vi "api_mqttInit.vi"(0 "client":string="LabVIEW_MQTT_Client", 5 "broker":T3={"address"="localhost", "port"=1883, "connTimeout"=2000, "writeTimeout"=2000, "readTimeout"=2000, "subTimeout"=30000}, 7 "connFlags":T2={"reserved"=FALSE, "clean session"=TRUE, "will flag"=TRUE, "willQOS"=enum."At most once", "will retain"=FALSE, "password"=FALSE, "user name"=FALSE}, 9 "User Info":T1={"User Name"="User", "Password"="password"}, 11 "error in (no error)":errorcluster) -> (4 "mqtt.lvclass out":refnum<class "mqtt.lvclass">, 10 "MQTT event":refnum<user-event>, 15 "error out":errorcluster)   [LabVIEW 2018, in "labview-mqtt.lvlib" / "mqtt.lvclass"]
uses:
  mqtt.lvclass
  mqttTypedef/mqttBroker.ctl
  mqttTypedef/mqttConnectionFlags.ctl
  mqttTypedef/mqttWillInformation.ctl
  mqttTypedef/mqttRXsubscriptionEventData.ctl
  mqtt.lvclass/mqtt.ctl
  labview-mqtt.lvlib
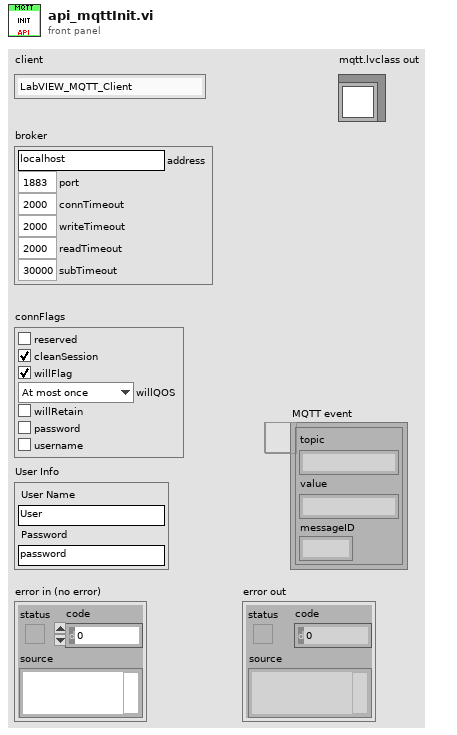
[diagram p1: front panel]
types:
  T1 = typedef "labview-mqtt.lvlib/mqttWillInformation.ctl" = cluster{"User Name":string, "Password":string}
  T2 = typedef "labview-mqtt.lvlib/mqttConnectionFlags.ctl" = cluster{"reserved":bool, "clean session":bool, "will flag":bool, "willQOS":enum8{"At most once", "At least once", "Exactly once", "Reserved"}, "will retain":bool, "password":bool, "user name":bool}
  T3 = typedef "labview-mqtt.lvlib/mqttBroker.ctl" = cluster{"address":string, "port":u16, "connTimeout":i32, "writeTimeout":i32, "readTimeout":i32, "subTimeout":i32}
  T4 = typedef "labview-mqtt.lvlib/mqttRXsubscriptionEventData.ctl" = cluster{"topic":string, "value":string, "messageID":u16}
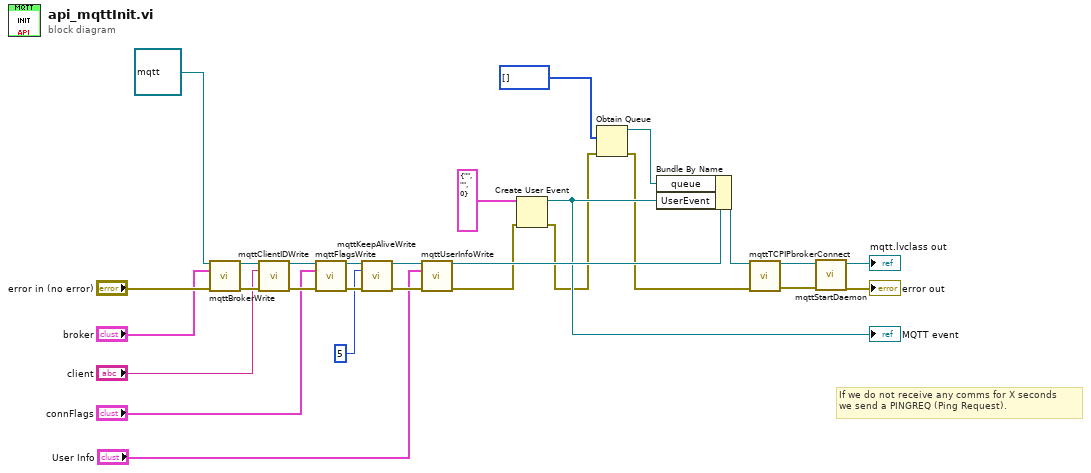
[diagram p0: block diagram]
diagram:
  # "If we do not receive any comms for X seconds\nwe send a PINGREQ (Ping Request)."
  n1 = call "mqttBrokerWrite.vi"("mqtt in"=refnum<class "mqtt.lvclass"> refnum ("mqtt.lvclass"), "broker"="broker", "error in (no error)"="error in (no error)") -> ("mqtt out"=w28:refnum<class "mqtt.lvclass">, "error out"=w27:errorcluster)  [unwired: 11 in]
  n2 = call "mqttClientIDWrite.vi"("mqtt in"=w28, "clientID"="client", "error in (no error)"=w27) -> ("mqtt out"=w23:refnum<class "mqtt.lvclass">, "error out"=w22:errorcluster)  [unwired: 11 in]
  n3 = call "mqttFlagsWrite.vi"("mqtt in"=w23, "connFlags"="connFlags", "error in (no error)"=w22) -> ("mqtt out"=w25:refnum<class "mqtt.lvclass">, "error out"=w24:errorcluster)  [unwired: 11 in]
  n4 = call "mqttKeepAliveWrite.vi"("mqtt in"=w25, "keepAlive(sec)"=u16 5, "error in (no error)"=w24) -> ("mqtt out"=w16:refnum<class "mqtt.lvclass">, "error out"=w15:errorcluster)  [unwired: 11 in]
  n5 = call "mqttUserInfoWrite.vi"("mqtt in"=w16, "User Info"="User Info", "error in (no error)"=w15) -> ("mqtt out"=w13:refnum<class "mqtt.lvclass">, "error out"=w11:errorcluster)  [unwired: 11 in]
  n6 = Create User Event(user event datatype=T4 {"topic"="", "value"="", "messageID"=0} ("data"), error in=w11) -> (user event=w10:refnum<user-event>, error out=w8:errorcluster)
  "MQTT event" <- w10
  n7 = Obtain Queue(element data type=u8[] [] ("telegram"), error in (no error)=w8) -> (queue out=w7:refnum<queue>, error out=w6:errorcluster)  [unwired: 3 in, 1 out]
  n8 = Bundle By Name(cluster=w13, "queue"=w7, "UserEvent"=w10) -> (w5:refnum<class "mqtt.lvclass">)
  n9 = call "mqttTCPIPbrokerConnect.vi"("mqtt in"=w5, "error in (no error)"=w6) -> ("mqtt out"=w4:refnum<class "mqtt.lvclass">, "error out"=w2:errorcluster)  [unwired: 12 in]
  n10 = call "mqttStartDaemon.vi"("error in (no error)"=w2, "mqtt in"=w4) -> ("error out"=→"error out":errorcluster, "mqtt out"=→"mqtt.lvclass out":refnum<class "mqtt.lvclass">)  [unwired: 8 in]
